vi "Read CAN Lookup.vi"(8 "error in (no error)":errorcluster, 11 "CAN Data in":refnum<class "CAN Data.lvclass">) -> (0 "error out":errorcluster, 2 "CAN Lookup":variant, 3 "CAN Data out":refnum<class "CAN Data.lvclass">)   [LabVIEW 2021, in "BS120x Driver.lvlib" / "Data Classes.lvlib" / "CAN Data.lvclass"]
uses:
  CAN Data.lvclass
  CAN Data.lvclass/CAN Data.ctl
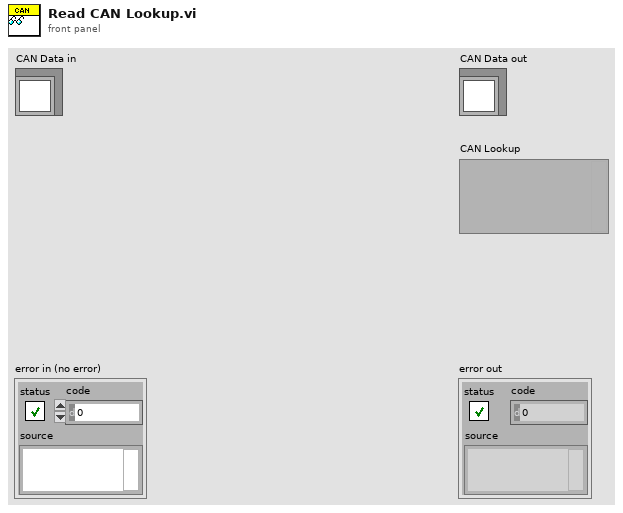
[diagram p1: front panel]
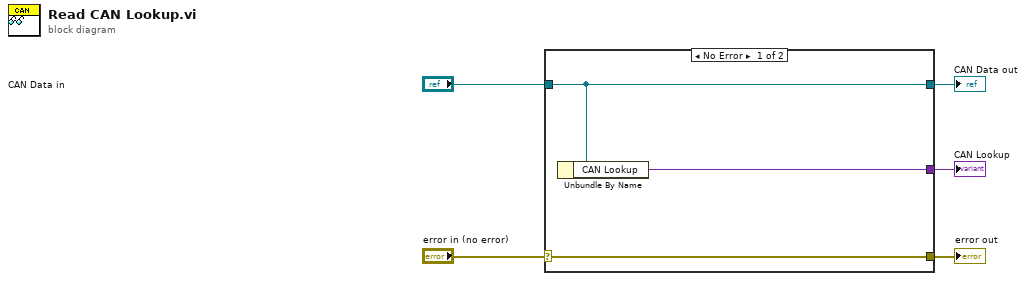
[diagram p0: block diagram]
diagram:
  n1 = case shown="No Error" "error in (no error)" {
    selector: "error in (no error)" -> [w8 w9]
    tunnel: [w8 w9] -> w4
    tunnel: [w7 w10] -> w2
    tunnel: "CAN Data in" -> [w7 w10]
    tunnel: [w6 _] -> w1
    frame No Error {
      n2 = Unbundle By Name(w7) -> ("CAN Lookup"=w6:variant)
    }
    frame Error {
    }
  }
  "error out" <- w4
  "CAN Data out" <- w2
  "CAN Lookup" <- w1
